vi "Data Viewer.vi"(0 "Path":path) -> ()   [LabVIEW 2012]
uses:
  <vilib>/Utility/NIReport.llb/NI_report.lvclass
  <vilib>/printing/ReportDocExtensions.llb/Append Front Panel Image to Report (path).vi
  <vilib>/Utility/config.llb/Write Key (Boolean).vi
  <vilib>/Utility/config.llb/NI_LVConfig.lvlib
  <vilib>/Utility/NIReport.llb/NI_ReportGenerationCore.lvlib
panel:
  out "TIC":bool
  in  "MR#":i32=1 caption="MR #"
  in  "Expt#":i32=1 caption="Expt #"
  in  "Link":bool=TRUE
  in  "Scan#":i32=1 caption="Scan #"
  in  "Avg":bool
  in  "Log":bool
  in  "CPS":bool
  out "Graph":cluster{"X":sgl[], "Y":sgl[]}(graph) caption="C:\\Users\\Min\\Projects\\Sniffer\\Build\\Data\\2 MRM d200 .isd"
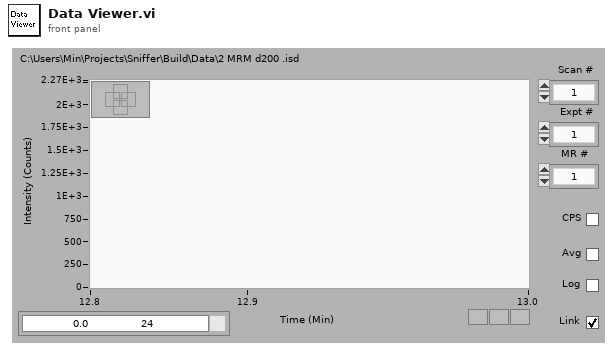
[diagram p1: front panel]
types:
  T1 = enum32{"existing file", "new file", "new or existing file", "existing dir", "new dir", "new or existing dir", "existing file (use LLBs)", "new file (use LLBs)", "new or existing file (use LLBs)", "new or existing file or directory (use LLBs)"}
  T2 = enum16{"Standard Report", "HTML", "Word", "Excel"}
  T3 = typedef "_Opion Switches.ctl" = cluster{"Averaging":bool, "Acquire":bool, "MCA":bool, "CPS":bool, "Log Scale":bool, "DC EN":bool, "DC POL":bool, "MRF EN":bool, "PS EN":bool}
  T4 = cluster{"left":i16, "top":i16, "right":i16, "bottom":i16}
  T5 = typedef "_Data.ctl" = cluster{"X":dbl[], "Y":dbl[], "Dwell Time (mS)":dbl, "X Title":string, "Time (s)":dbl, "TIC":u32, "# of Scans":i32, "Path":path, "ScanType":i32}
  T6 = cluster{"XScale.Minimum":dbl, "XScale.Maximum":dbl, "Cursor.Cursor X":dbl}
  T7 = typedef "LVRectTypeDef.ctl" = cluster{"Left":i16, "Top":i16, "Right":i16, "Bottom":i16}
  T8 = typedef "NI_LVConfig.lvlib/Config Data RefNum.ctl" = refnum<k1>
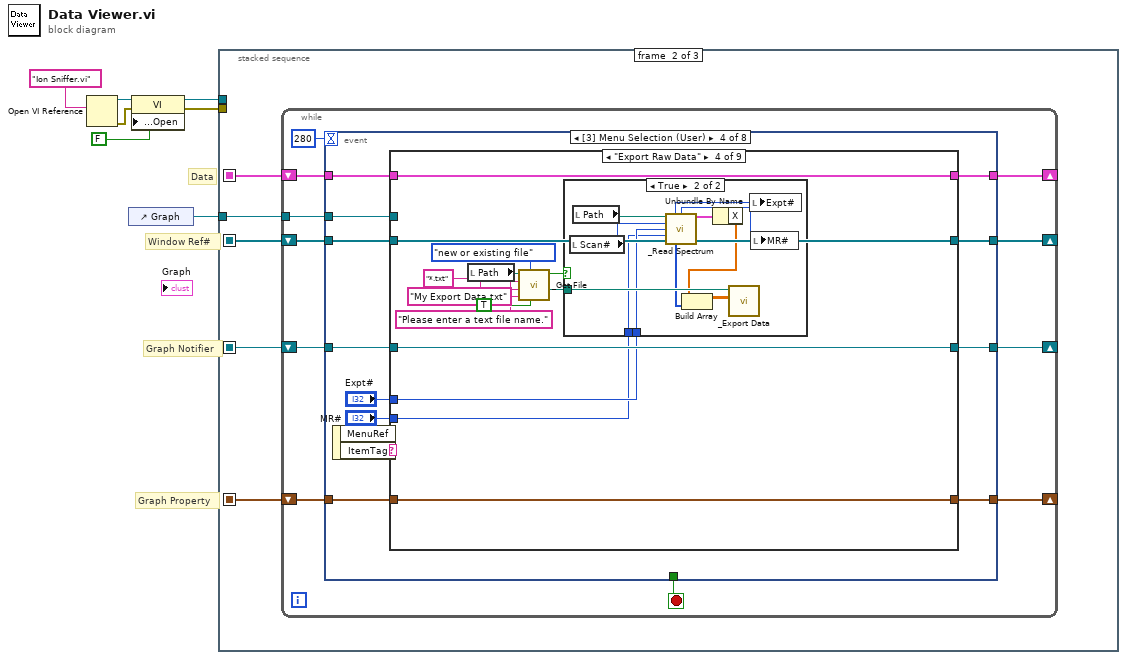
[diagram p0: block diagram]
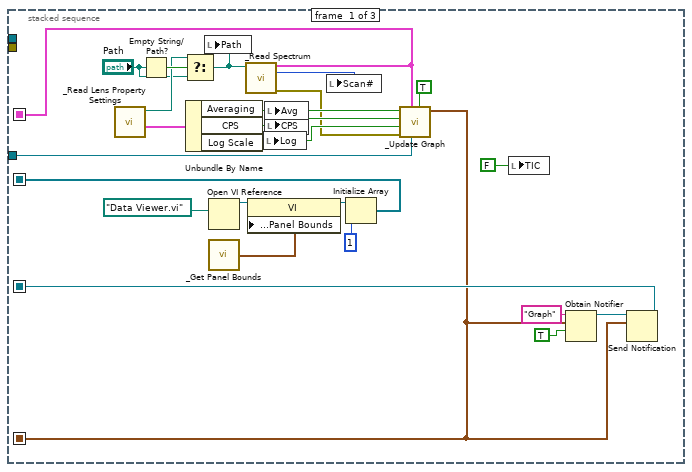
[diagram p2: hidden frame]
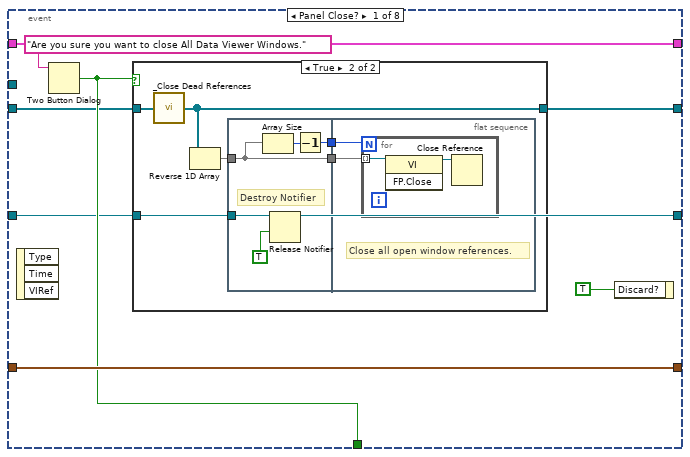
[diagram p3: hidden frame]
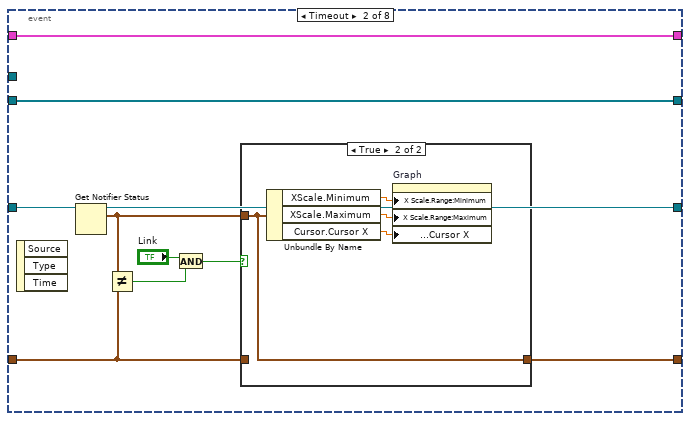
[diagram p5: hidden frame]
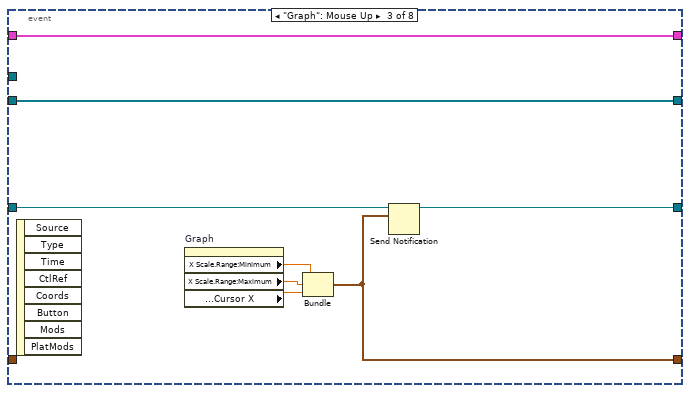
[diagram p7: hidden frame]
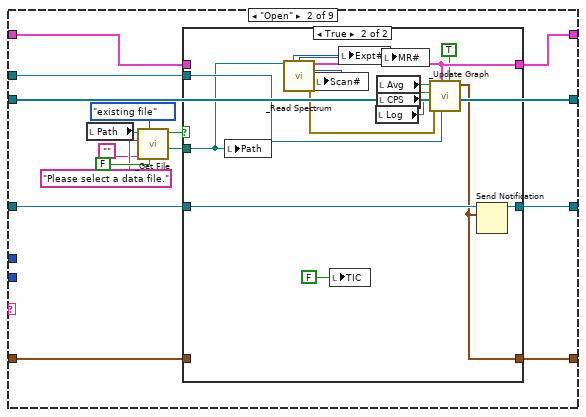
[diagram p9: hidden frame]
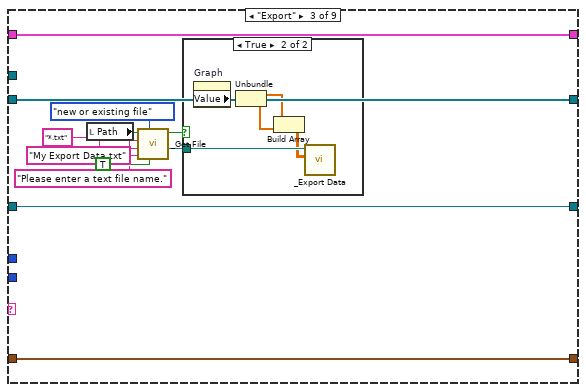
[diagram p11: hidden frame]
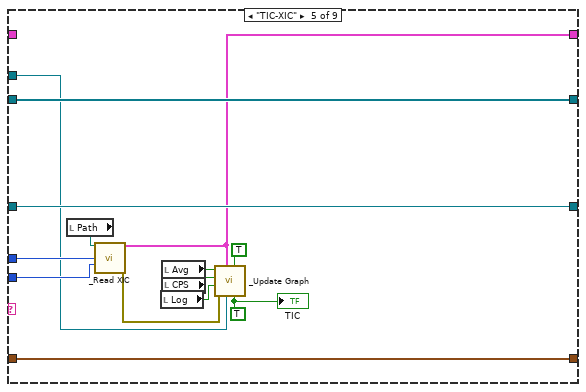
[diagram p14: hidden frame]
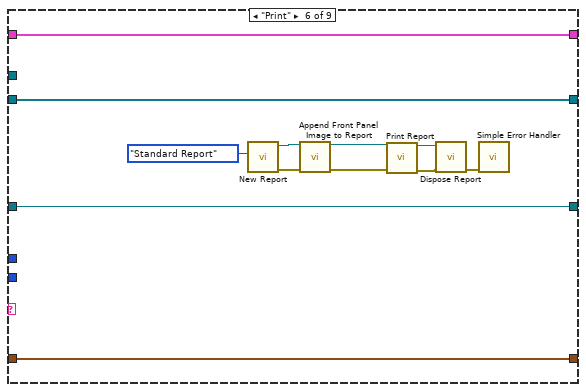
[diagram p15: hidden frame]
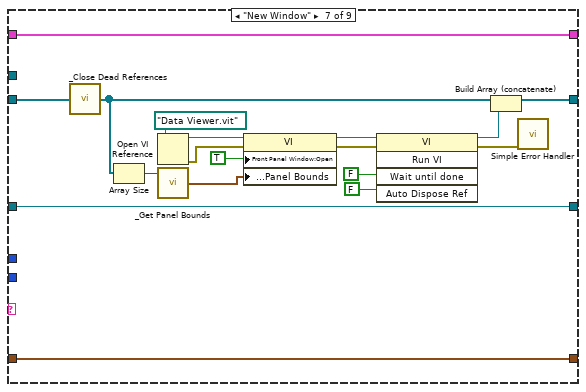
[diagram p16: hidden frame]
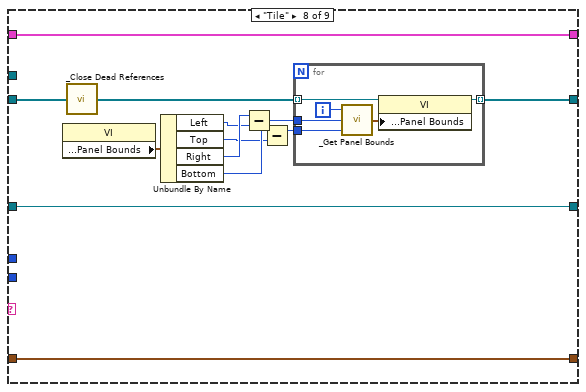
[diagram p17: hidden frame]
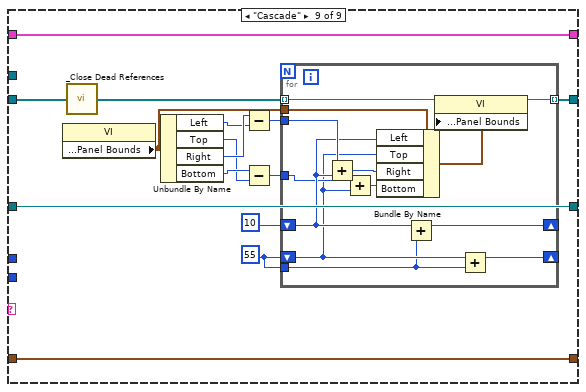
[diagram p18: hidden frame]
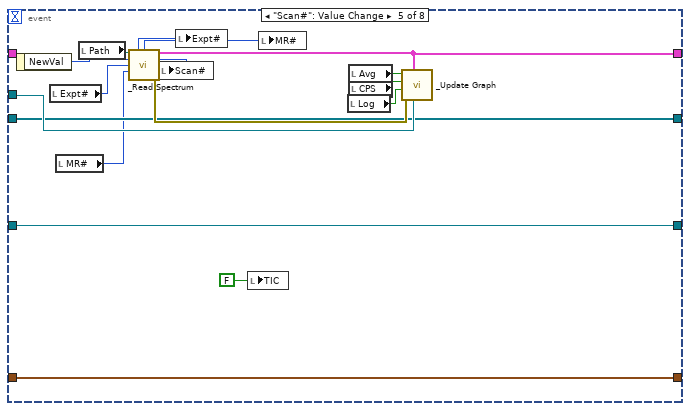
[diagram p19: hidden frame]
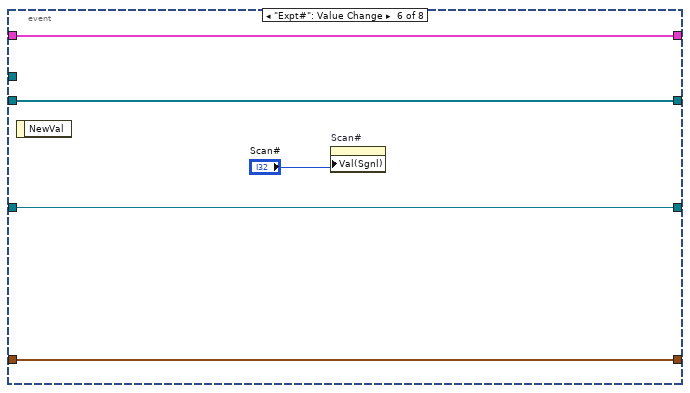
[diagram p20: hidden frame]
diagram:
  # "Data"
  # "Graph Notifier"
  # "Graph Property"
  # "Window Ref#"
  n1 = Open VI Reference(vi path="Ion Sniffer.vi") -> (vi reference=w5:refnum<vi>, error out=w4:errorcluster)  [unwired: 1 in, 4 out]
  n2 = control-ref of="Graph"() -> (w7:refnum<vi>)
  n3 = property class="VI"(reference=w5, error in=w4, "Front Panel Window:Open"=FALSE) -> (reference out=w2:refnum<vi>, error out=w1:errorcluster)
  n4 = stacked-sequence {
    seq-local: [w27 _ _] -> [_ w35 _]
    seq-local: [w24 _ _] -> [_ w37 _]
    seq-local: [w10 _ _] -> [_ w36 _]
    seq-local: [w12 _ _] -> [_ w34 _]
    tunnel: w7 -> [w11 w33 _]
    tunnel: w2 -> [_ _ w315]
    tunnel: w1 -> [_ _ w314]
    frame #0 {
      n5 = call "_Read Lens Property Settings.vi"() -> ("Switches"=w19:T3, "Spectrum File Path:"=w21:path)  [unwired: 6 out]
      n6 = Empty String/Path?(string/path="Path") -> (empty?=w22:bool)
      n7 = Select(t=w21, s=w22, f="Path") -> (s? t:f=w18:path)
      n8 = Unbundle By Name(w19) -> ("Averaging"=w16:bool, "CPS"=w15:bool, "Log Scale"=w14:bool)
      n9 = local write "Path"(w18) -> ()
      n10 = Open VI Reference(vi path=path "Data Viewer.vi") -> (vi reference=w29:refnum<vi>)  [unwired: 1 in, 5 out]
      n11 = call "_Get Panel Bounds.vi"() -> ("PanelBounds"=w28:T4)  [unwired: 3 in]
      n12 = call "_Read Spectrum.vi"("file path"=w18) -> ("Data"=w12:T5, "Scan# out"=w17:i32, "error out"=w13:errorcluster)  [unwired: 5 in, 7 out]
      n13 = property class="VI"(reference=w29, "Front Panel Window:Panel Bounds"=w28) -> (reference out=w31:refnum<vi>)  [unwired: 1 in, 1 out]
      n14 = local write "Log"(w14) -> ()
      n15 = local write "Avg"(w16) -> ()
      n16 = local write "CPS"(w15) -> ()
      n17 = local write "Scan#"(w17) -> ()
      n18 = Initialize Array(w31, 1 ("dimension size")) -> (w27:refnum<vi>[])
      n19 = call "_Update Graph.vi"("Auto Scale"=TRUE, "Graph Ref"=w11, "Data"=w12, "error in (no error)"=w13, "Log Scale"=w14, "CPS"=w15, "Averaging"=w16) -> ("Graph Property"=w10:T6)  [unwired: 1 in, 3 out]
      n20 = local write "TIC"(FALSE ("TIC")) -> ()
      n21 = Obtain Notifier(name (unnamed)="Graph", notification data type=w10, create if not found? (T)=TRUE) -> (notifier out=w26:refnum<notifier>)  [unwired: 1 in, 2 out]
      n22 = Send Notification(notification=w10, notifier=w26) -> (notifier out=w24:refnum<notifier>)  [unwired: 1 in, 1 out]
    }
    frame #1 {
      n23 = while {
        shift-right: [w46] -> _
        shift-left: w37 -> [w47]
        shift-right: [w44] -> _
        shift-left: w36 -> [w45]
        shift-right: [w42] -> _
        shift-left: w35 -> [w43]
        shift-right: [w39] -> _
        shift-left: w34 -> [w41]
        tunnel: w33 -> [w40]
        stop <- w48 stop-if-true
        n24 = event shown="[3] Menu Selection (User)" {
          selector: _ -> [_ _ _ _ _ _ _ _]
          dyn-events: _ -> [_ _ _ _ _ _ _ _]
          timeout: 280 -> [_ _ _ _ _ _ _ _]
          tunnel: [w53 _ _ _ _ _ _ _] -> w48
          tunnel: w47 -> [w51 w82 w95 w104 w284 w297 w302 w312]
          tunnel: [w51 w81 w94 w103 w284 w297 w302 w312] -> w46
          tunnel: w45 -> [w55 w80 _ w102 w283 w296 w301 w311]
          tunnel: [w55 w79 w91 w101 w283 w296 w301 w311] -> w44
          tunnel: w43 -> [w52 w77 w90 w106 w285 w298 w303 w313]
          tunnel: [w50 w77 w90 w105 w285 w298 w303 w313] -> w42
          tunnel: w41 -> [w49 w76 w89 w100 _ w299 w304 w306]
          tunnel: w40 -> [_ _ _ w98 w286 _ _ w307]
          tunnel: [w49 w76 w89 w99 w289 w299 w304 w306] -> w39
          event Panel Close? {
            n25 = event-data() -> ()  [unwired: 4 out]
            n26 = Two Button Dialog(message="Are you sure you want to close All Data Viewer Windows.") -> (T button?=w53:bool)  [unwired: 2 out]
            n27 = case shown="True" w53 {
              tunnel: w52 -> [w57 w63]
              tunnel: [w57 w62] -> w50
              tunnel: w51 -> [_ w61]
              frame False {
              }
              frame True {
                n28 = call "_Close Dead References.vi"("VI Ref Array In"=w63) -> ("VI Ref Array Out"=w62:refnum<vi>[])
                n29 = Reverse 1D Array(array=w62) -> (reversed array=w60:refnum<vi>[])
                n30 = flat-sequence {
                  tunnel: w61 -> [w67]
                  tunnel: w60 -> [w66]
                  tunnel: [w66] -> w59
                  tunnel: [w64] -> w58
                  tunnel: w59 -> [w70]
                  tunnel: w58 -> [w69]
                  frame #0 {
                    # "Destroy Notifier"
                    n31 = Array Size(array=w66) -> (size(s)=w65:i32)
                    n32 = Release Notifier(notifier=w67, force destroy? (F)=TRUE) -> ()  [unwired: 1 in, 3 out]
                    n33 = Decrement(x=w65) -> (x-1=w64:i32)
                  }
                  frame #1 {
                    # "Close all open window references."
                    n34 = for {
                      N: w69 -> [_]
                      tunnel: w70 -> [w71] mode=indexing
                      n35 = invoke class="VI" method="FP.Close"(reference=w71) -> (reference out=w72:refnum<vi>)  [unwired: 2 in, 2 out]
                      n36 = Close Reference(reference=w72) -> ()  [unwired: 1 in, 1 out]
                    }
                  }
                }
              }
            }
            n37 = event-data("Discard?"=TRUE) -> ()  [unwired: 1 in, 1 out]
          }
          event Timeout {
            n38 = event-data() -> ()  [unwired: 4 out]
            n39 = Get Notifier Status(notifier=w82) -> (notifier out=w81:refnum<notifier>, current notification=w78:T6)  [unwired: 1 in, 3 out]
            n40 = Not Equal?(x=w78, y=w80) -> (x != y?=w74:bool)
            n41 = And(x="Link", y=w74) -> (x .and. y?=w73:bool)
            n42 = case shown="True" w73 {
              tunnel: [w83 w84] -> w79
              tunnel: w80 -> [w83 _]
              tunnel: w78 -> [_ w84]
              frame False {
              }
              frame True {
                n43 = Unbundle By Name(w84) -> ("XScale.Minimum"=w87:dbl, "XScale.Maximum"=w86:dbl, "Cursor.Cursor X"=w85:dbl)
                n44 = property on="Graph" class="XYGraph (strict)"("X Scale.Range:Minimum"=w87, "X Scale.Range:Maximum"=w86, "Cursor.Cursor Position:Cursor X"=w85) -> ()  [unwired: 2 in, 2 out]
              }
            }
          }
          event "Graph": Mouse Up {
            n45 = event-data() -> ()  [unwired: 9 out]
            n46 = property on="Graph" class="XYGraph (strict)"() -> ("X Scale.Range:Minimum"=w93:dbl, "X Scale.Range:Maximum"=w92:dbl, "Cursor.Cursor Position:Cursor X"=w88:dbl)  [unwired: 2 in, 2 out]
            n47 = Bundle("XScale.Minimum"=w93, "XScale.Maximum"=w92, "Cursor.Cursor X"=w88) -> (w91:T6)  [unwired: 1 out]
            n48 = Send Notification(notification=w91, notifier=w95) -> (notifier out=w94:refnum<notifier>)  [unwired: 1 in, 1 out]
          }
          event Menu Selection (User) {
            n49 = event-data() -> ("ItemTag"=w107:string)  [unwired: 2 out]
            n50 = case shown="\"Export Raw Data\"" w107 {
              tunnel: w106 -> [w109 w126 w156 w175 w200 w211 w220 w241 w262]
              tunnel: [w109 w126 w156 w175 w200 w211 w218 w238 w259] -> w105
              tunnel: w104 -> [w111 w116 w147 w166 w199 w210 w230 w243 w264]
              tunnel: [w111 w115 w147 w166 w199 w210 w230 w243 w264] -> w103
              tunnel: [w110 w113 w146 w165 w198 w209 w229 w242 w263] -> w101
              tunnel: w102 -> [w110 w114 w146 w165 w198 w209 w229 w242 w263]
              tunnel: w100 -> [w108 w119 w145 w164 _ w212 w216 w240 w261]
              tunnel: [w108 w118 w145 w164 w189 w212 w216 w240 w261] -> w99
              tunnel: w98 -> [_ w117 _ _ w190 _ _ _ _]
              tunnel: "Expt#" -> [_ _ _ w163 w197 _ _ _ _]
              tunnel: "MR#" -> [_ _ _ w162 w196 _ _ _ _]
              frame Default {
              }
              frame "Open" {
                n51 = local read "Path"() -> (w125:path)
                n52 = call "_Get File.vi"("For Write (T)"=FALSE, "select mode (new or existing)"=T1."existing file", "default name"="", "prompt"="Please select a data file.", "Start Path"=w125) -> ("Seleted File"=w120:path, "Succeeded"=w121:bool)  [unwired: 1 in, 2 out]
                n53 = case shown="True" w121 {
                  tunnel: w120 -> [_ w137]
                  tunnel: w119 -> [w129 _]
                  tunnel: [w129 w139] -> w118
                  tunnel: w117 -> [_ w138]
                  tunnel: w116 -> [w127 w136]
                  tunnel: [w127 w135] -> w115
                  tunnel: [w128 w134] -> w113
                  tunnel: w114 -> [w128 _]
                  frame False {
                  }
                  frame True {
                    n54 = local write "Path"(w137) -> ()
                    n55 = call "_Read Spectrum.vi"("file path"=w137) -> ("Expt# Out"=w132:i32, "MR# Out"=w131:i32, "Data"=w139:T5, "Scan# out"=w144:i32, "error out"=w140:errorcluster)  [unwired: 5 in, 5 out]
                    n56 = local write "Scan#"(w144) -> ()
                    n57 = local write "TIC"(FALSE ("TIC")) -> ()
                    n58 = local write "Expt#"(w132) -> ()
                    n59 = local read "Log"() -> (w141:bool)
                    n60 = local read "Avg"() -> (w143:bool)
                    n61 = local read "CPS"() -> (w142:bool)
                    n62 = local write "MR#"(w131) -> ()
                    n63 = call "_Update Graph.vi"("Auto Scale"=TRUE, "Graph Ref"=w138, "Data"=w139, "error in (no error)"=w140, "Log Scale"=w141, "CPS"=w142, "Averaging"=w143) -> ("Graph Property"=w134:T6)  [unwired: 1 in, 3 out]
                    n64 = Send Notification(notification=w134, notifier=w136) -> (notifier out=w135:refnum<notifier>)  [unwired: 1 in, 1 out]
                  }
                }
              }
              frame "Export" {
                n65 = local read "Path"() -> (w155:path)
                n66 = call "_Get File.vi"("For Write (T)"=TRUE, "select mode (new or existing)"=T1."new or existing file", "default name"="My Export Data.txt", "extension (isd)"="*.txt", "prompt"="Please enter a text file name.", "Start Path"=w155) -> ("Seleted File"=w150:path, "Succeeded"=w151:bool)  [unwired: 2 out]
                n67 = case shown="True" w151 {
                  tunnel: w150 -> [_ w161]
                  frame False {
                  }
                  frame True {
                    n68 = property on="Graph" class="XYGraph (strict)"() -> ("Value"=w159:cluster{"X":sgl[], "Y":sgl[]})  [unwired: 2 in, 2 out]
                    n69 = Unbundle(w159) -> ("X"=w158:sgl[], "Y"=w157:sgl[])
                    n70 = Build Array(w158, w157) -> (w160:sgl[][])
                    n71 = call "_Export Data.vi"("2D data"=w160, "file path (dialog if empty)"=w161) -> ()  [unwired: 1 in, 6 out]
                  }
                }
              }
              frame "Export Raw Data" {
                n72 = local read "Path"() -> (w174:path)
                n73 = call "_Get File.vi"("For Write (T)"=TRUE, "select mode (new or existing)"=T1."new or existing file", "default name"="My Export Data.txt", "extension (isd)"="*.txt", "prompt"="Please enter a text file name.", "Start Path"=w174) -> ("Seleted File"=w169:path, "Succeeded"=w170:bool)  [unwired: 2 out]
                n74 = case shown="True" w170 {
                  tunnel: w169 -> [_ w186]
                  tunnel: w163 -> [_ w179]
                  tunnel: w162 -> [_ w177]
                  frame False {
                  }
                  frame True {
                    n75 = local read "Scan#"() -> (w183:i32)
                    n76 = local read "Path"() -> (w184:path)
                    n77 = call "_Read Spectrum.vi"("file path"=w184, "Scan# (1-based)"=w183, "Expt# (1-based)"=w179, "MR# (1-based)"=w177) -> ("Expt# Out"=w178:i32, "MR# Out"=w176:i32, "Data"=w182:T5, "raw data"=w180:i32[])  [unwired: 2 in, 6 out]
                    n78 = Unbundle By Name(w182) -> ("X"=w181:dbl[])
                    n79 = Build Array(w181, w180) -> (w185:dbl[][])
                    n80 = call "_Export Data.vi"("2D data"=w185, "file path (dialog if empty)"=w186) -> ()  [unwired: 1 in, 6 out]
                    n81 = local write "Expt#"(w178) -> ()
                    n82 = local write "MR#"(w176) -> ()
                  }
                }
              }
              frame "TIC-XIC" {
                w187 = TRUE ("TIC (F)")
                n83 = local read "Path"() -> (w195:path)
                n84 = call "_Read XIC.vi"("file path"=w195, "Expt#"=w197, "MR#"=w196) -> ("Data"=w189:T5, "error out"=w188:errorcluster)  [unwired: 1 in, 10 out]
                n85 = local read "Log"() -> (w192:bool)
                n86 = local read "Avg"() -> (w194:bool)
                n87 = local read "CPS"() -> (w193:bool)
                n88 = call "_Update Graph.vi"("TIC (F)"=w187, "Auto Scale"=TRUE, "Graph Ref"=w190, "Data"=w189, "error in (no error)"=w188, "Log Scale"=w192, "CPS"=w193, "Averaging"=w194) -> ()  [unwired: 4 out]
                "TIC" <- w187
              }
              frame "Print" {
                n89 = call <vilib>:"New Report.vi"("report type"=T2."Standard Report") -> ("report out"=w205:refnum<class "NI_report.lvclass">, "error out"=w206:errorcluster)  [unwired: 5 in, 8 out]
                n90 = call-poly <vilib>:"Append Front Panel Image to Report.vi"("report in"=w205, "error in (no error)"=w206) -> ("report out"=w207:refnum<class "NI_report.lvclass">, "error out"=w208:errorcluster)  [unwired: 6 in, 6 out]
                n91 = call-dynamic "Print Report.vi"("report in"=w207, "error in (no error)"=w208) -> ("report out"=w203:refnum<class "NI_report.lvclass">, "error out"=w204:errorcluster)  [unwired: 2 in, 10 out]
                n92 = call-dynamic "Dispose Report.vi"("report in"=w203, "error in (no error)"=w204) -> ("error out"=w202:errorcluster)  [unwired: 3 in, 10 out]
                n93 = call <vilib>:"Simple Error Handler.vi"("error in (no error)"=w202) -> ()  [unwired: 1 in, 8 out]
              }
              frame "New Window" {
                n94 = call "_Close Dead References.vi"("VI Ref Array In"=w220) -> ("VI Ref Array Out"=w213:refnum<vi>[])
                n95 = Array Size(array=w213) -> (size(s)=w214:i32)
                n96 = Open VI Reference(vi path=path "Data Viewer.vit") -> (vi reference=w225:refnum<vi>, error out=w222:errorcluster)  [unwired: 1 in, 4 out]
                n97 = call "_Get Panel Bounds.vi"("Zero-based Panel #"=w214) -> ("PanelBounds"=w217:T4)  [unwired: 2 in]
                n98 = property class="VI"(reference=w225, error in=w222, "Front Panel Window:Open"=TRUE, "Front Panel Window:Panel Bounds"=w217) -> (reference out=w223:refnum<vi>, error out=w221:errorcluster)
                n99 = invoke class="VI" method="Run VI"(reference=w223, error in=w221, "Wait until done"=FALSE, "Auto Dispose Ref"=FALSE) -> (reference out=w219:refnum<vi>, error out=w215:errorcluster)  [unwired: 1 in, 3 out]
                n100 = Build Array (concatenate)(w213, w219) -> (w218:refnum<vi>[])
                n101 = call <vilib>:"Simple Error Handler.vi"("error in (no error)"=w215) -> ()  [unwired: 1 in, 8 out]
              }
              frame "Tile" {
                n102 = property class="VI"() -> ("Front Panel Window:Panel Bounds"=w237:T7)  [unwired: 2 in, 2 out]
                n103 = call "_Close Dead References.vi"("VI Ref Array In"=w241) -> ("VI Ref Array Out"=w239:refnum<vi>[])
                n104 = Unbundle By Name(w237) -> ("Left"=w235:i16, "Top"=w232:i16, "Right"=w236:i16, "Bottom"=w233:i16)
                n105 = Subtract(x=w236, y=w235) -> (x-y=w234:i16)
                n106 = Subtract(x=w233, y=w232) -> (x-y=w231:i16)
                n107 = for {
                  tunnel: w239 -> [w248] mode=indexing
                  tunnel: [w247] -> w238 mode=indexing
                  tunnel: w234 -> [w245]
                  tunnel: w231 -> [w244]
                  i -> [w246]
                  n108 = call "_Get Panel Bounds.vi"("Panel Height"=w244, "Panel Width"=w245, "Zero-based Panel #"=w246) -> ("PanelBounds"=w249:T4)
                  n109 = property class="VI"(reference=w248, "Front Panel Window:Panel Bounds"=w249) -> (reference out=w247:refnum<vi>)  [unwired: 1 in, 1 out]
                }
              }
              frame "Cascade" {
                w251 = i16 55 ("bottom")
                n110 = property class="VI"() -> ("Front Panel Window:Panel Bounds"=w250:T7)  [unwired: 2 in, 2 out]
                n111 = call "_Close Dead References.vi"("VI Ref Array In"=w262) -> ("VI Ref Array Out"=w260:refnum<vi>[])
                n112 = Unbundle By Name(w250) -> ("Left"=w257:i16, "Top"=w254:i16, "Right"=w258:i16, "Bottom"=w255:i16)
                n113 = Subtract(x=w258, y=w257) -> (x-y=w256:i16)
                n114 = Subtract(x=w255, y=w254) -> (x-y=w253:i16)
                n115 = for {
                  tunnel: w260 -> [w277] mode=indexing
                  tunnel: [w276] -> w259 mode=indexing
                  tunnel: w256 -> [w271]
                  tunnel: w253 -> [w267]
                  shift-right: [w274] -> _
                  shift-left: i16 10 ("bottom") -> [w270]
                  shift-right: [w273] -> _
                  shift-left: w251 -> [w266]
                  tunnel: w251 -> [w265]
                  tunnel: w250 -> [w272]
                  n116 = Add(x=w271, y=w270) -> (x+y=w269:i16)
                  n117 = Add(x=w267, y=w266) -> (x+y=w268:i16)
                  n118 = Bundle By Name(cluster=w272, "Left"=w270, "Top"=w266, "Right"=w269, "Bottom"=w268) -> (w275:T7)
                  n119 = Add(x=w270, y=w265) -> (x+y=w274:i16)
                  n120 = property class="VI"(reference=w277, "Front Panel Window:Panel Bounds"=w275) -> (reference out=w276:refnum<vi>)  [unwired: 1 in, 1 out]
                  n121 = Add(x=w266, y=w265) -> (x+y=w273:i16)
                }
              }
            }
          }
          event "Scan#": Value Change {
            n122 = event-data() -> ("NewVal"=w287:i32)  [unwired: 1 out]
            n123 = local read "Expt#"() -> (w281:i32)
            n124 = local read "MR#"() -> (w280:i32)
            n125 = local read "Path"() -> (w294:path)
            n126 = call "_Read Spectrum.vi"("file path"=w294, "Scan# (1-based)"=w287, "Expt# (1-based)"=w281, "MR# (1-based)"=w280) -> ("Expt# Out"=w282:i32, "MR# Out"=w279:i32, "Data"=w289:T5, "Scan# out"=w293:i32, "error out"=w288:errorcluster)  [unwired: 2 in, 5 out]
            n127 = local write "Scan#"(w293) -> ()
            n128 = local write "Expt#"(w282) -> ()
            n129 = local write "TIC"(FALSE ("TIC")) -> ()
            n130 = local write "MR#"(w279) -> ()
            n131 = local read "Log"() -> (w290:bool)
            n132 = local read "Avg"() -> (w292:bool)
            n133 = local read "CPS"() -> (w291:bool)
            n134 = call "_Update Graph.vi"("Graph Ref"=w286, "Data"=w289, "error in (no error)"=w288, "Log Scale"=w290, "CPS"=w291, "Averaging"=w292) -> ()  [unwired: 2 in, 4 out]
          }
          event "Expt#": Value Change {
            n135 = event-data() -> ()  [unwired: 2 out]
            n136 = property on="Scan#" class="DigNum (strict)"("Val(Sgnl)"="Scan#") -> ()  [unwired: 2 in, 2 out]
          }
          event "MR#": Value Change {
            n137 = event-data() -> ()  [unwired: 2 out]
            n138 = local read "Scan#"() -> (w300:i32)
            n139 = property on="Scan#" class="DigNum (strict)"("Val(Sgnl)"=w300) -> ()  [unwired: 2 in, 2 out]
          }
          event "CPS", "Log", "Avg": Value Change {
            n140 = event-data() -> ()  [unwired: 7 out]
            n141 = local read "TIC"() -> (w305:bool)
            n142 = call "_Update Graph.vi"("TIC (F)"=w305, "Graph Ref"=w307, "Data"=w306, "Log Scale"="Log", "CPS"="CPS", "Averaging"="Avg") -> ()  [unwired: 2 in, 4 out]
          }
        }
      }
    }
    frame #2 {
      w328 = "Lens" ("section")
      n143 = property class="VI"(reference=w315, error in=w314, "Front Panel Window:Open"=TRUE) -> (reference out=w316:refnum<vi>, error out=w317:errorcluster)
      n144 = Close Reference(reference=w316, error in (no error)=w317) -> ()  [unwired: 1 out]
      n145 = local read "Avg"() -> (w321:bool)
      n146 = local read "CPS"() -> (w320:bool)
      n147 = local read "Log"() -> (w319:bool)
      n148 = call "_Open Preference File.vi"() -> ("error"=w322:errorcluster, "refnum"=w327:T8)  [unwired: 1 in, 5 out]
      n149 = call-poly <vilib>:"Write Key.vi"("section"=w328, "error in (no error)"=w322, "value"=w321, "key"="Averaging" ("section"), "refnum"=w327) -> ("error out"=w323:errorcluster, "refnum out"=w326:T8)  [unwired: 5 out]
      n150 = call-poly <vilib>:"Write Key.vi"("section"=w328, "error in (no error)"=w323, "value"=w320, "key"="CPS" ("section"), "refnum"=w326) -> ("error out"=w331:errorcluster, "refnum out"=w330:T8)  [unwired: 5 out]
      n151 = call-poly <vilib>:"Write Key.vi"("section"=w328, "error in (no error)"=w331, "value"=w319, "key"="LogScale" ("section"), "refnum"=w330) -> ("error out"=w324:errorcluster, "refnum out"=w325:T8)  [unwired: 5 out]
      n152 = call <vilib>:"Close Config Data.vi"("error in (no error)"=w324, "refnum"=w325) -> ()  [unwired: 1 in, 9 out]
    }
  }
